vi "continuous_cam.vi"() -> ()   [LabVIEW 2023]
doc: "This example demonstrates how to call a Python function and pass integers as arguments. It uses a python function to compute the sum of two integers."
uses:
  Program Files (x86)/National Instruments/LabVIEW 2021/examples/Connectivity/Python/support/PythonVersionsEnum.ctl
panel:
  out "error out":errorcluster
  in  "error in (no error)":errorcluster
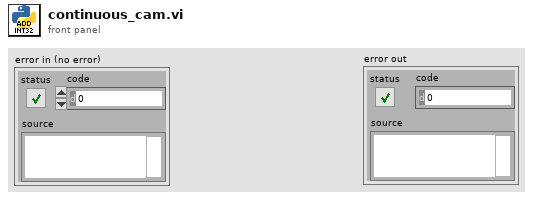
[diagram p1: front panel]
types:
  T1 = typedef "PythonVersionsEnum.ctl" = enum16{"3.6", "3.7", "3.8", "3.9"}
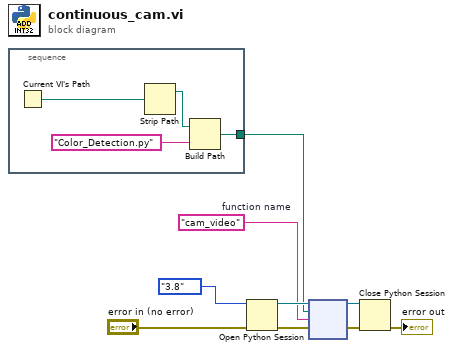
[diagram p0: block diagram]
diagram:
  w5 = "cam_video"  # function name
  n1 = stacked-sequence {
    tunnel: [w13] -> w6
    frame #0 {
      n2 = Current VI's Path() -> (path=w10:path)
      n3 = Strip Path(path=w10) -> (stripped path=w11:path)  [unwired: 1 out]
      n4 = Build Path(base path=w11, name or relative path="Color_Detection.py") -> (appended path=w13:path)
    }
  }
  n5 = Open Python Session(python version=PythonVersionsEnum."3.8", 3:"error in (no error)") -> (session out=w8:refnum<k35>, error out=w7:errorcluster)  [unwired: 1 in]
  n6 = node(w8, w6, w5, w7) -> (w4:refnum<k35>, w3:errorcluster)  [unwired: 2 in, 2 out]
  n7 = Close Python Session(session in=w4, error in=w3) -> (11:→"error out":errorcluster)
